vi "Joystick_Control.vi"() -> ()   [LabVIEW 2017]
uses:
  TypeDefs/JoystickControls.ctl
panel:
  in  "Joystick control":T1
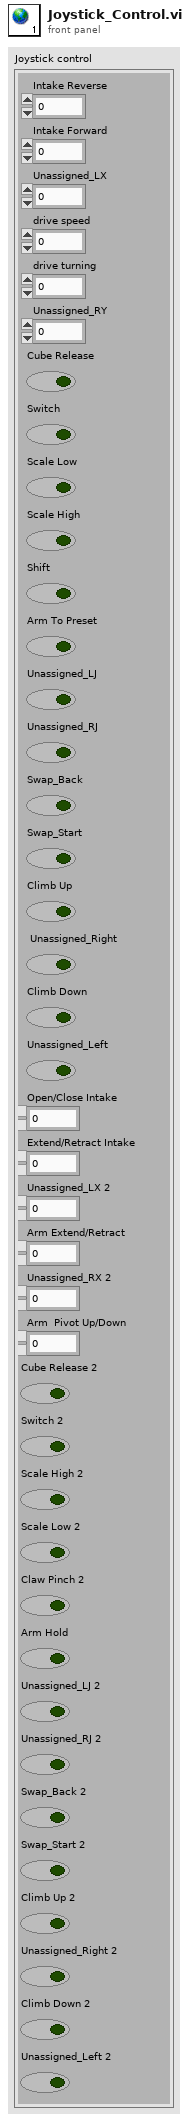
[diagram p1: front panel]
types:
  T1 = typedef "JoystickControls.ctl" = cluster{"drive speed":dbl, "drive turning":dbl, "Unassigned_LX":dbl, "Unassigned_RY":dbl, "Cube Release":bool, "Intake Forward":dbl, "Intake Reverse ":dbl, "Switch":bool, "Scale Low":bool, "Scale High":bool, "Shift":bool, "Arm To Preset":bool, "Unassigned_LJ":bool, "Unassigned_RJ":bool, "Swap_Back":bool, "Swap_Start":bool, "Arm Extend/Retract":dbl, "Unassigned_RX 2":dbl, "Unassigned_LX 2":dbl, "Arm  Pivot Up/Down ":dbl, "Cube Release 2":bool, "Extend/Retract Intake":dbl, "Open/Close Intake":dbl, "Switch 2":bool, "Scale High 2":bool, "Scale Low 2":bool, "Claw Pinch 2":bool, "Arm Hold":bool, "Unassigned_LJ 2":bool, "Unassigned_RJ 2":bool, "Swap_Back 2":bool, "Swap_Start 2":bool, "Climb Up 2":bool, "Unassigned_Right 2":bool, "Climb Down 2":bool, "Unassigned_Left 2":bool, "Climb Up ":bool, " Unassigned_Right":bool, "Climb Down":bool, "Unassigned_Left":bool}
diagram:
